vi "Set UI Loop References.vi"(7 "UI Data in":T1={"SR Display List"=[], "Filter Cluster"={"Show Resolved"=TRUE, "Show Potentially Resolved"=TRUE, "Show Passoffs"=TRUE, "Show In Collab"=TRUE}, "Exit"=refnum, "Main VI"=refnum, "Sorting"=enum."SR Status", "Message"=refnum, "Legend"=refnum, "Sorting Reference"=refnum, "SR Display List Reference"=refnum, "Filter Cluster Reference"=refnum} {"SR Display List"."Creation Date" format="%<%x>T"; "SR Display List"."Last Updated" format="%<%x>T"}, 8 "error in":errorcluster, 11 "call chain":string[](array[string])) -> (0 "error out":errorcluster, 1 "UI Data out":T1={"SR Display List"=[], "Filter Cluster"={"Show Resolved"=TRUE, "Show Potentially Resolved"=TRUE, "Show Passoffs"=TRUE, "Show In Collab"=TRUE}, "Exit"=refnum, "Main VI"=refnum, "Sorting"=enum."SR Status", "Message"=refnum, "Legend"=refnum, "Sorting Reference"=refnum, "SR Display List Reference"=refnum, "Filter Cluster Reference"=refnum} {"SR Display List"."Creation Date" format="%<%x>T"; "SR Display List"."Last Updated" format="%<%x>T"})   [LabVIEW 2018]
doc: "Pulls needed front panel references and bundles them into the UI data cluster"
uses:
  Type Defs/UI Loop Data.ctl
  Type Defs/SR Cluster.ctl
  Type Defs/SR Status.ctl
  Type Defs/Filter Cluster.ctl
  Type Defs/Sorting Methods.ctl
  Type Defs/SR Display List Reference.ctl
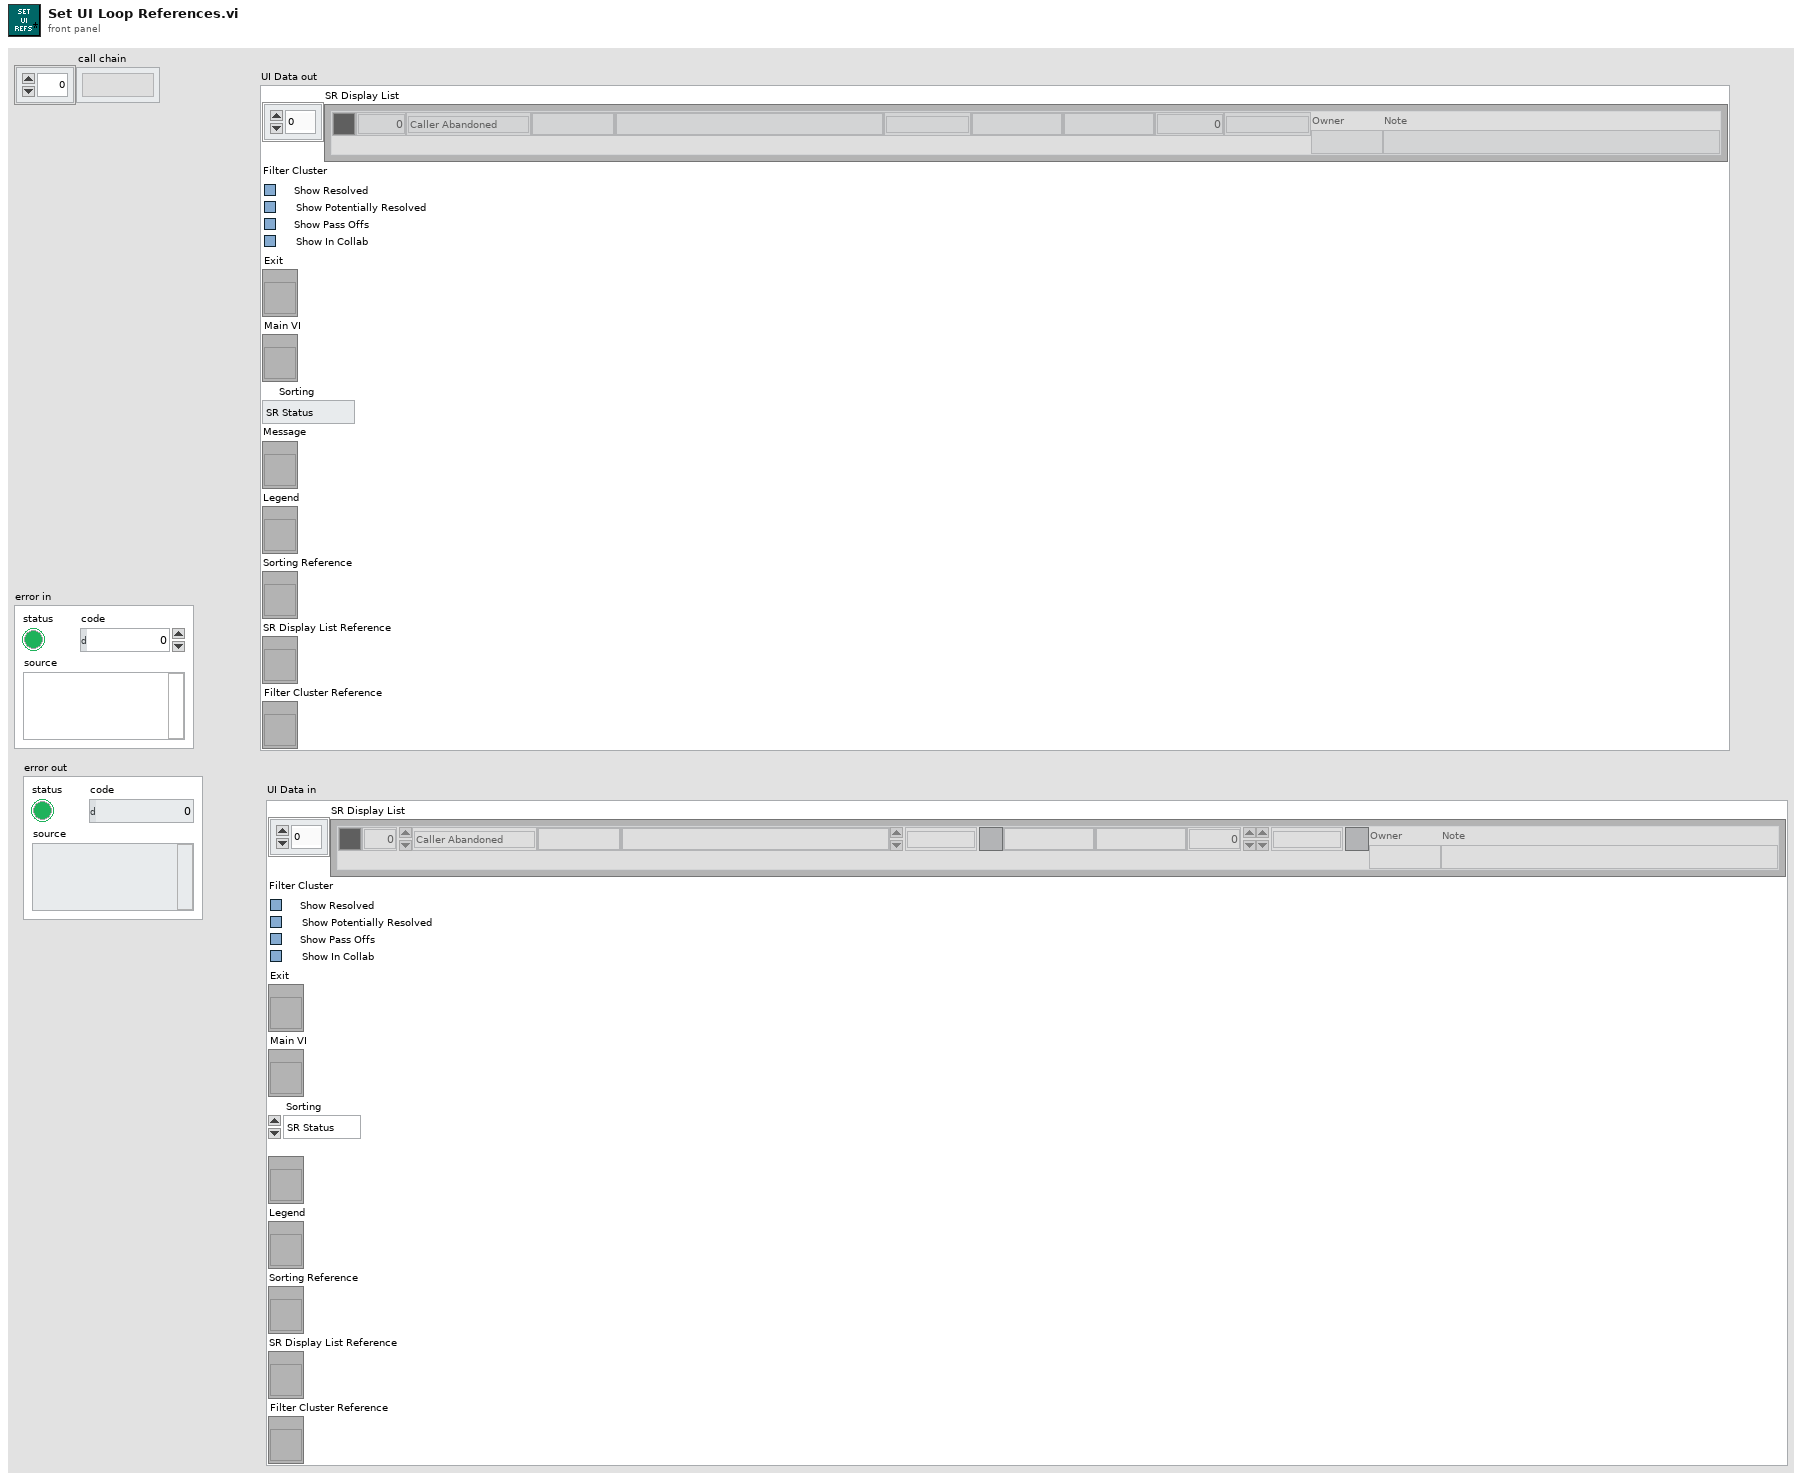
[diagram p1: front panel]
types:
  T1 = typedef "UI Loop Data.ctl" = cluster{"SR Display List":T2[], "Filter Cluster":T4, "Exit":refnum<vi>, "Main VI":refnum<vi>, "Sorting":T5, "Message":refnum<vi>, "Legend":refnum<vi>, "Sorting Reference":refnum<vi>, "SR Display List Reference":T6, "Filter Cluster Reference":refnum<vi>}
  T2 = typedef "SR Cluster.ctl" = cluster{"Color":u32, "SR Number":i32, "SR Status":T3, "Name":string, "Summary":string, "Last Updated":timestamp, "SR Type":string, "Service Level":string, "Days Open":dbl, "Creation Date":timestamp, "Owner":string, "Note":string}
  T3 = typedef "SR Status.ctl" = enum16{"Caller Abandoned", "Created in Error", "Expired", "Forum Resolved AE", "Forum Resolved Customer", "IN WORK", "IN WORK Collab with AES", "IN WORK Collab with PSE", "IN WORK Collab with SE", "IN WORK Customer Added Note", "IN WORK Escalation", "IN WORK Wait on Customer", "Open", "Potentially Resolved", "Presumed Resolved", "RMA Approved for Return", "RMA Closed", "RMA Closed - DOA", "RMA In Progress", "RMA Open", "RMA Waiting on Customer", "Resolved", "Passed Off"}
  T4 = typedef "Filter Cluster.ctl" = cluster{"Show Resolved":bool, "Show Potentially Resolved":bool, "Show Passoffs":bool, "Show In Collab":bool}
  T5 = typedef "Sorting Methods.ctl" = enum16{"SR Status", "Most Recent", "SR Type", "SR Number", "Days Open", "Urgency"}
  T6 = typedef "SR Display List Reference.ctl" = refnum<vi>
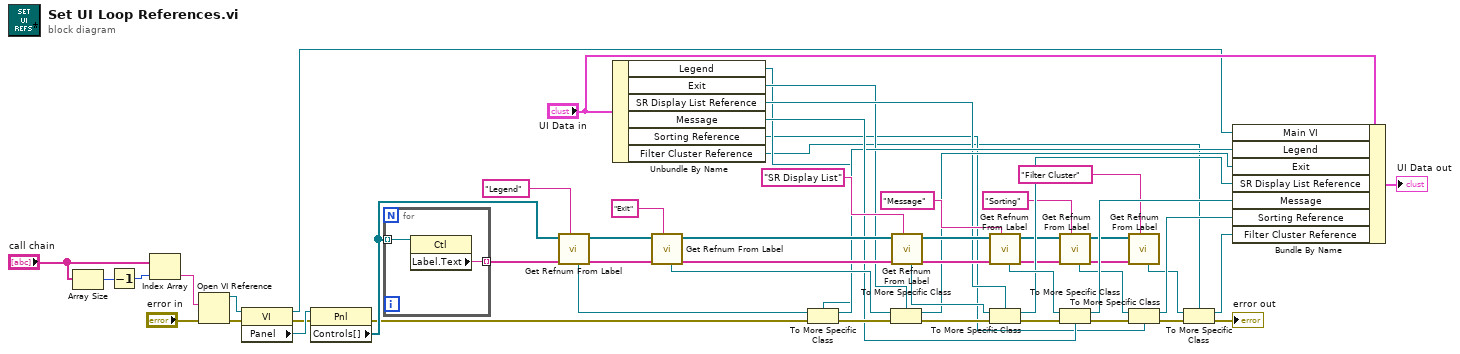
[diagram p0: block diagram]
diagram:
  n1 = Array Size(array="call chain") -> (size(s)=w39:i32)
  n2 = Decrement(x=w39) -> (x-1=w40:i32)
  n3 = Index Array(array="call chain", index=w40) -> (element=w41:string)
  n4 = Open VI Reference(vi path=w41, error in (no error)="error in") -> (vi reference=w55:refnum<vi>, error out=w50:errorcluster)  [unwired: 4 in]
  n5 = property class="VI"(reference=w55, error in=w50) -> (reference out=w33:refnum<vi>, error out=w51:errorcluster, "Panel"=w52:refnum<vi>)
  n6 = property class="Pnl"(reference=w52, error in=w51) -> (error out=w24:errorcluster, "Controls[]"=w29:refnum<vi>[])  [unwired: 1 out]
  n7 = for {
    tunnel: w29 -> [w57] mode=indexing
    tunnel: [w56] -> w28 mode=indexing
    n8 = property class="Ctl"(reference=w57) -> ("Label.Text"=w56:string)  [unwired: 1 in, 2 out]
  }
  n9 = call "Get Refnum From Label.vi"("label"="Legend", "label array in"=w28, "controls[] in"=w29) -> ("label array out"=w27:string[], "controls[] out"=w30:refnum<vi>[], "refnum out"=w26:refnum<vi>)  [unwired: 6 in]
  n10 = Unbundle By Name("UI Data in") -> ("Legend"=w16:refnum<vi>, "Exit"=w17:refnum<vi>, "SR Display List Reference"=w18:T6, "Message"=w23:refnum<vi>, "Sorting Reference"=w15:refnum<vi>, "Filter Cluster Reference"=w6:refnum<vi>)
  n11 = call "Get Refnum From Label.vi"("label"="Exit", "label array in"=w27, "controls[] in"=w30) -> ("label array out"=w44:string[], "controls[] out"=w43:refnum<vi>[], "refnum out"=w45:refnum<vi>)  [unwired: 6 in]
  n12 = To More Specific Class(target class=w16, reference=w26, error in=w24) -> (specific class reference=w19:refnum<vi>, error out=w25:errorcluster)
  n13 = To More Specific Class(target class=w17, reference=w45, error in=w25) -> (specific class reference=w20:refnum<vi>, error out=w47:errorcluster)
  n14 = call "Get Refnum From Label.vi"("label"="SR Display List", "label array in"=w44, "controls[] in"=w43) -> ("label array out"=w36:string[], "controls[] out"=w37:refnum<vi>[], "refnum out"=w48:refnum<vi>)  [unwired: 6 in]
  n15 = call "Get Refnum From Label.vi"("label"="Message", "label array in"=w36, "controls[] in"=w37) -> ("label array out"=w13:string[], "controls[] out"=w14:refnum<vi>[], "refnum out"=w35:refnum<vi>)  [unwired: 6 in]
  n16 = To More Specific Class(target class=w18, reference=w48, error in=w47) -> (specific class reference=w21:T6, error out=w34:errorcluster)
  n17 = call "Get Refnum From Label.vi"("label"="Sorting", "label array in"=w13, "controls[] in"=w14) -> ("label array out"=w3:string[], "controls[] out"=w5:refnum<vi>[], "refnum out"=w4:refnum<vi>)  [unwired: 6 in]
  n18 = To More Specific Class(target class=w23, reference=w35, error in=w34) -> (specific class reference=w22:refnum<vi>, error out=w11:errorcluster)
  n19 = call "Get Refnum From Label.vi"("label"="Filter Cluster", "label array in"=w3, "controls[] in"=w5) -> ("refnum out"=w2:refnum<vi>)  [unwired: 6 in, 2 out]
  n20 = To More Specific Class(target class=w15, reference=w4, error in=w11) -> (specific class reference=w10:refnum<vi>, error out=w9:errorcluster)
  n21 = To More Specific Class(target class=w6, reference=w2, error in=w9) -> (specific class reference=w7:refnum<vi>, error out=→"error out":errorcluster)
  n22 = Bundle By Name(cluster="UI Data in", "Main VI"=w33, "Legend"=w19, "Exit"=w20, "SR Display List Reference"=w21, "Message"=w22, "Sorting Reference"=w10, "Filter Cluster Reference"=w7) -> (→"UI Data out":T1)
